vi "Excel_Set_Scale.vi"(0 "Axes in":refnum<k7>, 5 "Type":i32(ring)=1 items=["xlCategory"=1, "xlSeriesAxis"=3, "xlValue"=2], 11 "error in (no error)":errorcluster, 12 "axis config":T1={"autoscale"=FALSE, "min"=0.0, "max"=0.0, "scale type"=-4132} {"scale type" items=["xlScaleLinear"=-4132, "xlScaleLogarithmic"=-4133]; "max" format="%0.2f"; "min" format="%0.2f"}) -> (4 "Axes out":refnum<k7>, 15 "error out":errorcluster)   [LabVIEW 2017, in "NI_ReportGenerationToolkit.lvlib"]
uses:
  <vilib>/addons/_office/NI_ReportGenerationToolkit.lvlib
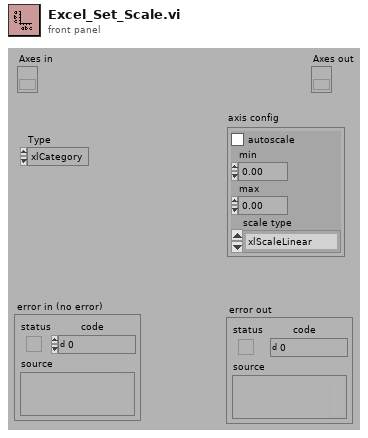
[diagram p1: front panel]
types:
  T1 = cluster{"autoscale":bool, "min":dbl, "max":dbl, "scale type":i32}
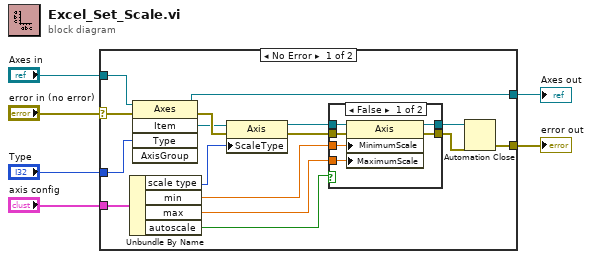
[diagram p0: block diagram]
diagram:
  n1 = case shown="No Error" "error in (no error)" {
    selector: "error in (no error)" -> [w7 w31]
    tunnel: [w22 w32] -> w6
    tunnel: "Axes in" -> [w20 w32]
    tunnel: "Type" -> [w17 _]
    tunnel: "axis config" -> [w16 _]
    tunnel: [w9 w31] -> w2
    frame No Error {
      n2 = Unbundle By Name(w16) -> ("scale type"=w21:i32, "min"=w12:dbl, "max"=w11:dbl, "autoscale"=w10:bool)
      n3 = invoke class="Axes" method="Item"(reference=w20, error in=w7, "Type"=w17) -> (reference out=w22:refnum<k7>, error out=w19:errorcluster, "Item"=w18:refnum<k7>)  [unwired: 2 in, 2 out]
      n4 = property class="Axis"(reference=w18, error in=w19, "ScaleType"=w21) -> (reference out=w15:refnum<k7>, error out=w13:errorcluster)
      n5 = case shown="False" w10 {
        tunnel: w15 -> [w28 w30]
        tunnel: [w27 w30] -> w14
        tunnel: w13 -> [w26 w29]
        tunnel: [w25 w29] -> w8
        tunnel: w12 -> [w24 _]
        tunnel: w11 -> [w23 _]
        frame False {
          n6 = property class="Axis"(reference=w28, error in=w26, "MinimumScale"=w24, "MaximumScale"=w23) -> (reference out=w27:refnum<k7>, error out=w25:errorcluster)
        }
        frame True {
        }
      }
      n7 = Automation Close(3:w8, 5:w14) -> (0:w9:errorcluster)
    }
    frame Error {
    }
  }
  "error out" <- w2
  "Axes out" <- w6
